vi "Read DataBlocks.vi"(0 "TCP Network Connection in":refnum<k5>, 1 "DBW LETTURE":T2(array[cluster]), 2 "DB REAL LETTURE":T1(array[cluster]), 3 "DB BIT LETTURE":cluster{"DB":i16, "BIT":i16[], "DBoffset":i16}[](array[cluster]), 5 "error in (no error)":errorcluster) -> (14 "TCP Network Connection out":refnum<k5>, 16 "DB WORD":dbl[](array[numeric]), 17 "DB REAL":dbl[](array[numeric]), 18 "Array DB bit":bool[](array[boolean]), 19 "error out":errorcluster)   [LabVIEW 2019]
uses:
  SIEMENS/S7Com_Source/S7Com_Data_Array.ctl
  SIEMENS/S7Com_Source/S7Com_RW_CMD.ctl
  SIEMENS/S7Com_Source/S7Com_Address_Area.ctl
  SIEMENS/S7Com_Source/S7Com_Start_Add.ctl
  SIEMENS/S7Com_Source/S7Com_Transport_Size.ctl
  SIEMENS/S7Com_Source/S7Com_Function.ctl
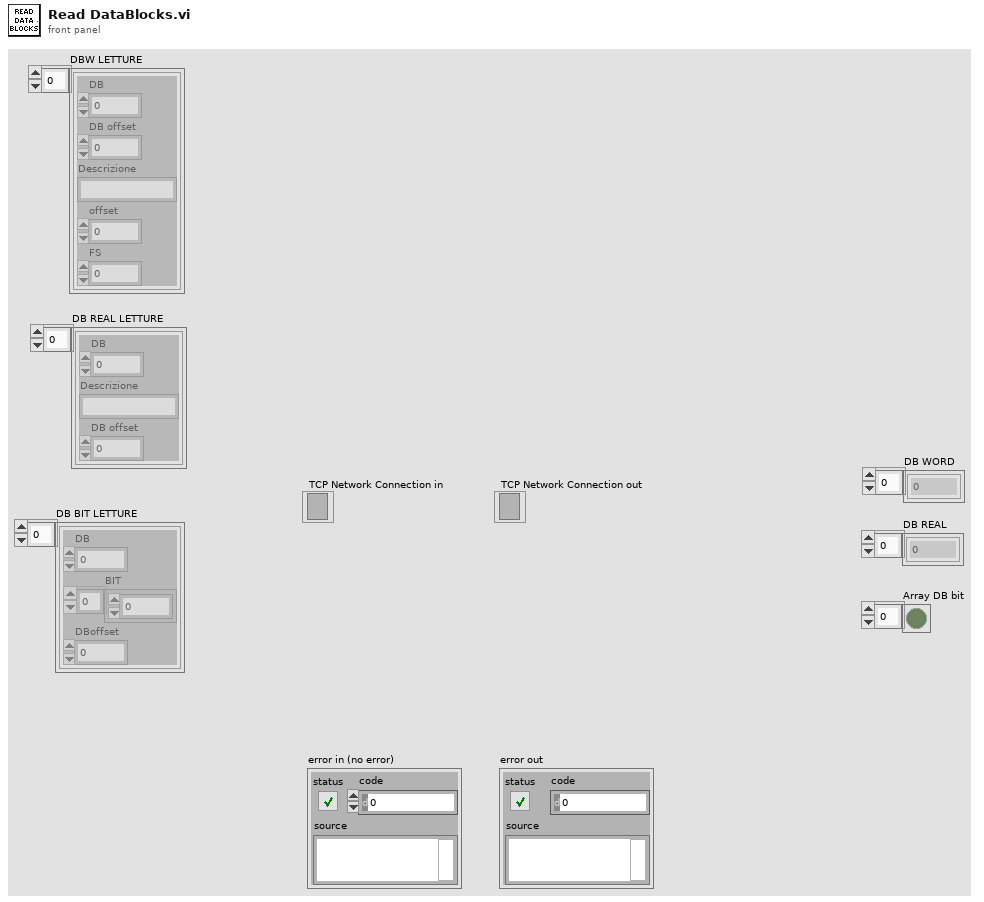
[diagram p1: front panel]
types:
  T1 = cluster{"DB":i16, "Descrizione":string, "DB offset":i16}[]
  T2 = cluster{"DB":i16, "DB offset":i16, "Descrizione":string, "offset":dbl, "FS":dbl}[]
  T3 = typedef "S7Com_Data_Array.ctl" = i32[]
  T4 = typedef "S7Com_RW_CMD.ctl" = cluster{"Read Length":u16, "Data Block #":u16, "S7_Add_Area":T5, "Start Address":T6, "S7_Transport_Size":T7, "S7_Function":T8}
  T5 = typedef "S7Com_Address_Area.ctl" = u8
  T6 = typedef "S7Com_Start_Add.ctl" = u16
  T7 = typedef "S7Com_Transport_Size.ctl" = u8
  T8 = typedef "S7Com_Function.ctl" = u8
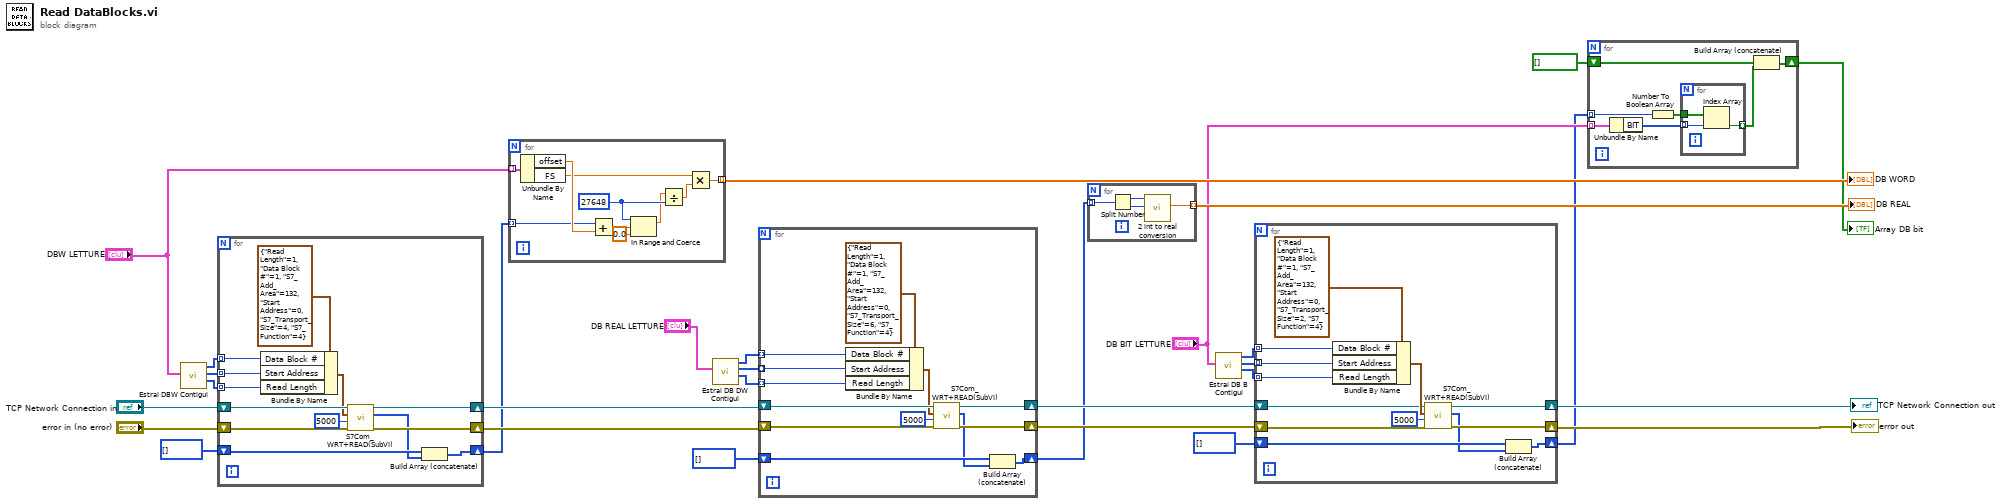
[diagram p0: block diagram]
diagram:
  n1 = call "Estrai DBW Contigui.vi"("DBW LETTURE"="DBW LETTURE") -> ("DBW number"=w19:i32[], "DB offset"=w20:i32[], "DB"=w21:i16[])  [unwired: 8 in]
  n2 = for {
    shift-right: [w40] -> w27
    shift-left: "error in (no error)" -> [w41]
    shift-right: [w42] -> w28
    shift-left: "TCP Network Connection in" -> [w43]
    tunnel: w21 -> [w37] mode=indexing
    tunnel: w20 -> [w36] mode=indexing
    tunnel: w19 -> [w34] mode=indexing
    shift-right: [w32] -> w17
    shift-left: T3 [] ("Read_Data") -> [w33]
    n3 = Bundle By Name(cluster=T4 {"Read Length"=1, "Data Block #"=1, "S7_Add_Area"=132, "Start Address"=0, "S7_Transport_Size"=4, "S7_Function"=4} ("RW_CMD"), "Data Block #"=w37, "Start Address"=w36, "Read Length"=w34) -> (w39:T4)
    n4 = call "S7Com_WRT+READ(SubVI).vi"("error in"=w41, "timeout ms (25000)"=5000, "RW_CMD"=w39, "connection ID in"=w43) -> ("error out"=w40:errorcluster, "Read_Data"=w31:T3, "connection ID out"=w42:refnum<k5>)  [unwired: 1 in, 1 out]
    n5 = Build Array (concatenate)(w33, w31) -> (w32:T3)
  }
  n6 = for {
    tunnel: "DBW LETTURE" -> [w53] mode=indexing
    tunnel: [w49] -> w16 mode=indexing
    tunnel: w17 -> [w44] mode=indexing
    w46 = 27648 ("y")
    n7 = Unbundle By Name(w53) -> ("offset"=w52:dbl, "FS"=w50:dbl)
    n8 = Add(x=w44, y=w52) -> (x+y=w48:dbl)
    n9 = In Range and Coerce(upper limit=w46, x=w48, lower limit=0.0) -> (coerced(x)=w45:dbl)  [unwired: 1 out]
    n10 = Divide(x=w45, y=w46) -> (x/y=w51:dbl)
    n11 = Multiply(x=w50, y=w51) -> (x*y=w49:dbl)
  }
  "DB WORD" <- w16
  n12 = call "Estrai DB DW Contigui.vi"("DB REAL LETTURE"="DB REAL LETTURE") -> ("DBW number"=w12:i32[], "DB offset"=w13:i32[], "DB"=w14:i16[])  [unwired: 8 in]
  n13 = for {
    shift-right: [w62] -> w25
    shift-left: w27 -> [w63]
    shift-right: [w64] -> w26
    shift-left: w28 -> [w65]
    tunnel: w14 -> [w59] mode=indexing
    tunnel: w13 -> [w58] mode=indexing
    tunnel: w12 -> [w57] mode=indexing
    shift-right: [w54] -> w10
    shift-left: T3 [] ("Read_Data") -> [w56]
    n14 = Bundle By Name(cluster=T4 {"Read Length"=1, "Data Block #"=1, "S7_Add_Area"=132, "Start Address"=0, "S7_Transport_Size"=6, "S7_Function"=4} ("RW_CMD"), "Data Block #"=w59, "Start Address"=w58, "Read Length"=w57) -> (w61:T4)
    n15 = call "S7Com_WRT+READ(SubVI).vi"("error in"=w63, "timeout ms (25000)"=5000, "RW_CMD"=w61, "connection ID in"=w65) -> ("error out"=w62:errorcluster, "Read_Data"=w55:T3, "connection ID out"=w64:refnum<k5>)  [unwired: 1 in, 1 out]
    n16 = Build Array (concatenate)(w56, w55) -> (w54:T3)
  }
  n17 = for {
    tunnel: [w68] -> w9 mode=indexing
    tunnel: w10 -> [w67] mode=indexing
    n18 = Split Number(x=w67) -> (hi(x)=w70:u16, lo(x)=w69:u16)
    n19 = call "2 int to real conversion.vi"("MW 15 0 in"=w69, "MW 31 16 in"=w70) -> ("reale out"=w68:dbl)  [unwired: 7 in, 2 out]
  }
  "DB REAL" <- w9
  n20 = call "Estrai DB B Contigui.vi"("DB BIT LETTURE"="DB BIT LETTURE") -> ("DB B number"=w4:i32[], "DB offset"=w5:i32[], "DB"=w6:i16[])  [unwired: 8 in]
  n21 = for {
    shift-right: [w78] -> w24
    shift-left: w25 -> [w79]
    shift-right: [w80] -> w23
    shift-left: w26 -> [w81]
    tunnel: w6 -> [w76] mode=indexing
    tunnel: w5 -> [w75] mode=indexing
    tunnel: w4 -> [w74] mode=indexing
    shift-right: [w71] -> w1
    shift-left: T3 [] ("Read_Data") -> [w73]
    n22 = Bundle By Name(cluster=T4 {"Read Length"=1, "Data Block #"=1, "S7_Add_Area"=132, "Start Address"=0, "S7_Transport_Size"=2, "S7_Function"=4} ("RW_CMD"), "Data Block #"=w76, "Start Address"=w75, "Read Length"=w74) -> (w83:T4)
    n23 = call "S7Com_WRT+READ(SubVI).vi"("error in"=w79, "timeout ms (25000)"=5000, "RW_CMD"=w83, "connection ID in"=w81) -> ("error out"=w78:errorcluster, "Read_Data"=w72:T3, "connection ID out"=w80:refnum<k5>)  [unwired: 1 in, 1 out]
    n24 = Build Array (concatenate)(w73, w72) -> (w71:T3)
  }
  "TCP Network Connection out" <- w23
  "error out" <- w24
  n25 = for {
    tunnel: "DB BIT LETTURE" -> [w90] mode=indexing
    shift-right: [w85] -> w2
    shift-left: bool[] [] -> [w86]
    tunnel: w1 -> [w84] mode=indexing
    n26 = Unbundle By Name(w90) -> ("BIT"=w89:i16[])
    n27 = Number To Boolean Array(number=w84) -> (Boolean array=w88:bool[])
    n28 = for {
      tunnel: w89 -> [w93] mode=indexing
      tunnel: w88 -> [w92]
      tunnel: [w91] -> w87 mode=indexing
      n29 = Index Array(array=w92, index=w93) -> (element=w91:bool)
    }
    n30 = Build Array (concatenate)(w86, w87) -> (w85:bool[])
  }
  "Array DB bit" <- w2
